vi "Simulator DMM Calibrate.vi"(8 "error in (no error)":errorcluster, 10 "Normalization Off? (F)":bool) -> (0 "error out":errorcluster {"code" format="%.0x"}, 3 "Normalization":T1)   [LabVIEW 2011]
uses:
  DMM Normalization State.ctl
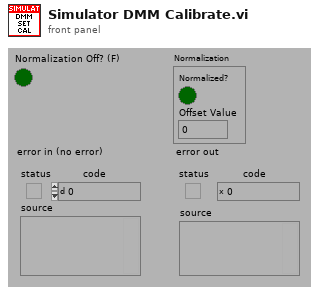
[diagram p1: front panel]
types:
  T1 = typedef "DMM Normalization State.ctl" = cluster{"Normalized?":bool, "Offset Value":dbl}
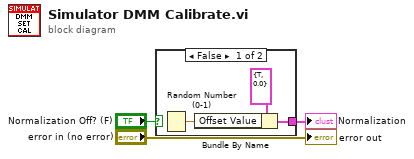
[diagram p0: block diagram]
diagram:
  n1 = case shown="False" "Normalization Off? (F)" {
    tunnel: [w4 _] -> w1
    frame False {
      n2 = Random Number (0-1)() -> (number: 0 to 1=w5:dbl)
      n3 = Bundle By Name(cluster=T1 {"Normalized?"=TRUE, "Offset Value"=0.0} ("Normalization"), "Offset Value"=w5) -> (w4:T1)
    }
    frame True {
    }
  }
  "Normalization" <- w1
  "error out" <- "error in (no error)"
